vi "Write Product Name.vi"(8 "error in (no error)":errorcluster, 10 "Product Name":string, 11 "PostBuildSupport in":refnum<class "PostBuildSupport.lvclass">) -> (0 "error out":errorcluster, 3 "PostBuildSupport out":refnum<class "PostBuildSupport.lvclass">)   [LabVIEW 2016, in "PostBuildSupport.lvclass"]
uses:
  PostBuildSupport.lvclass
  PostBuildSupport.lvclass/PostBuildSupport.ctl
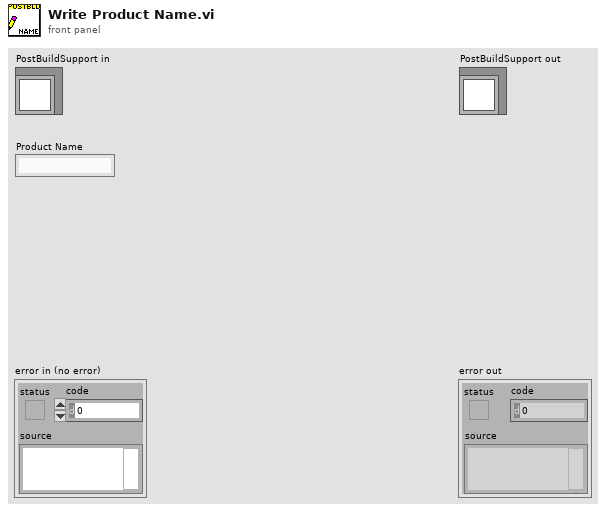
[diagram p1: front panel]
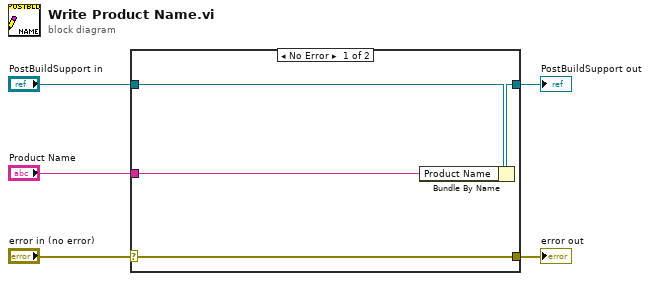
[diagram p0: block diagram]
diagram:
  n1 = case shown="No Error" "error in (no error)" {
    selector: "error in (no error)" -> [w9 w10]
    tunnel: [w9 w10] -> w4
    tunnel: [w7 w11] -> w2
    tunnel: "PostBuildSupport in" -> [w8 w11]
    tunnel: "Product Name" -> [w6 _]
    frame No Error {
      n2 = Bundle By Name(cluster=w8, "Product Name"=w6) -> (w7:refnum<class "PostBuildSupport.lvclass">)
    }
    frame Error {
    }
  }
  "error out" <- w4
  "PostBuildSupport out" <- w2
